vi "AlazarGetCPLDVersion.vi"(0 "Handle":u64, 11 "error in (no error)":errorcluster) -> (4 "Handle":u64, 6 "Major":u8, 8 "Minor":u8, 10 "Return Code":u32, 15 "error out":errorcluster)   [LabVIEW 2009]
doc: "Get the CPLD version number of the specified board."
uses:
  ATSApi.dll
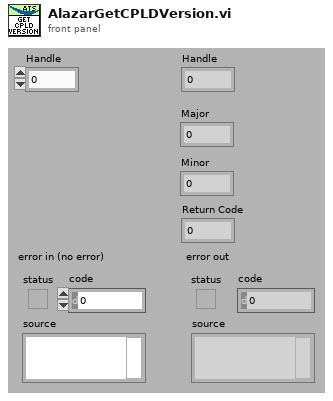
[diagram p1: front panel]
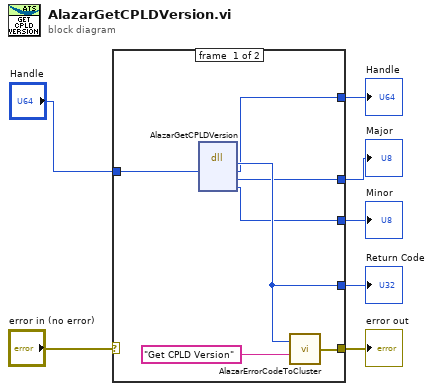
[diagram p0: block diagram]
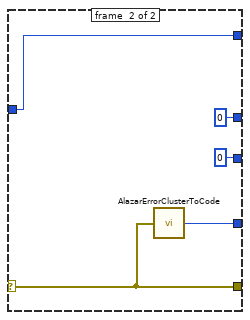
[diagram p2: hidden frame]
diagram:
  n1 = case shown="No Error" "error in (no error)" {
    selector: "error in (no error)" -> [_ w19]
    tunnel: [w11 w19] -> w6
    tunnel: [w13 w18] -> w5
    tunnel: "Handle" -> [w14 w17]
    tunnel: [w10 w17] -> w3
    tunnel: [w9 0] -> w2
    tunnel: [w8 0] -> w1
    frame #0 {
      n2 = dll-call lib="ATSApi.dll" fn="AlazarGetCPLDVersion"("handle"=w14) -> ("return type"=w13:u32, "handle"=w10:u64, "major"=w9:u8, "minor"=w8:u8)  [unwired: 5 in, 2 out]
      n3 = call "AlazarErrorCodeToCluster.vi"("Message"="Get CPLD Version", "Error Code"=w13) -> ("error out"=w11:errorcluster)
    }
    frame #1 {
      n4 = call "AlazarErrorClusterToCode.vi"("error in (no error)"=w19) -> ("Error Code"=w18:u32)
    }
  }
  "Handle" <- w3
  "error out" <- w6
  "Return Code" <- w5
  "Minor" <- w1
  "Major" <- w2
